vi "Read Forces.vi"(8 "error in":errorcluster, 10 "index":i32, 11 "CIFCorePlugin in":refnum<class "CIFCorePlugin.lvclass">) -> (0 "error out":errorcluster, 2 "Force":T1 {"Force Data" format="%x"}, 3 "CIFCorePlugin out":refnum<class "CIFCorePlugin.lvclass">)   [LabVIEW 2021, in "CIFCorePlugin.lvclass"]
uses:
  CIFCorePlugin.lvclass
  Common/Typedef/Channel Force Data.ctl
  CIFCorePlugin.lvclass/CIFCorePlugin.ctl
  Common/CIFCoreCommon.lvlib
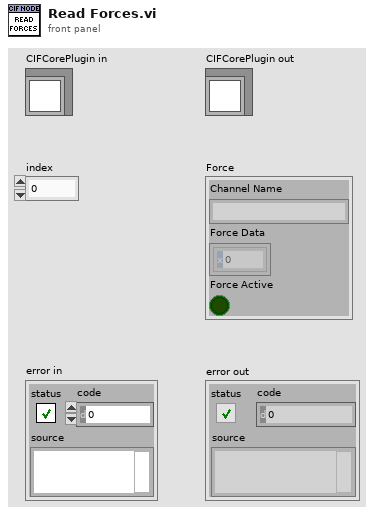
[diagram p1: front panel]
types:
  T1 = typedef "CIFCoreCommon.lvlib/Channel Force Data.ctl" = cluster{"Channel Name":string, "Force Data":u8[], "Force Active":bool}
  T2 = typedef "CIFCorePlugin.lvclass/gRPC to Main DVR.ctl" = refnum<data-value>
  T3 = typedef "CIFCoreCommon.lvlib/gRPC to Main Data.ctl" = cluster{"Config Data":variant, "Connections":T4[], "Forces":T1[], "Clock Conversion":T5, "Publisher Instance":T7}
  T4 = typedef "CIFCoreCommon.lvlib/Channel Connection Data.ctl" = cluster{"Publisher Name":string, "Subscriber Name":string, "Connection Data":u8[]}
  T5 = typedef "Time_CIF_U.lvlib/Clock Conversion Map.ctl" = map{u8, cluster{"Last Reset":i64, "Offset Pair":T6, "Slope":dbl, "1/Slope":dbl}}
  T6 = typedef "Time_CIF_U.lvlib/Timestamp Pair.ctl" = cluster{"System Time":i64, "External Time":i64}
  T7 = typedef "CIFCoreCommon.lvlib/FIFO Publisher.ctl" = cluster{"Publisher Name":string, "New FIFO Instance Config":T8}
  T8 = typedef "ChannelCommon.lvlib/New FIFO Instance Configuration.ctl" = cluster{"Backpressure":bool, "Bytes/Message Override":u32, "Messages/FIFO Override":u32, "Custom Data":u8[]}
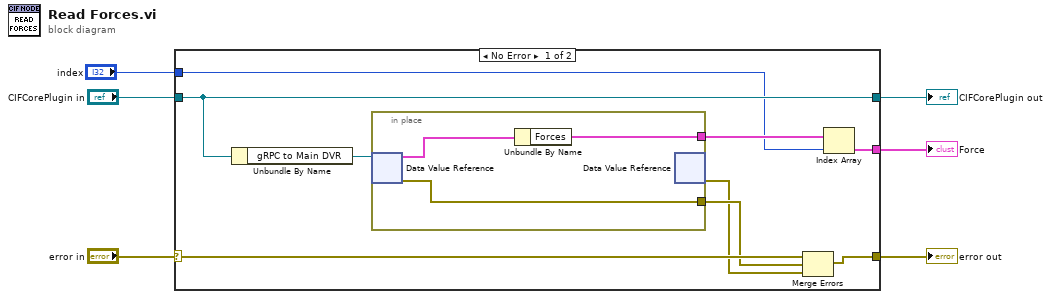
[diagram p0: block diagram]
diagram:
  n1 = case shown="No Error" "error in" {
    selector: "error in" -> [w13 w20]
    tunnel: [w10 w20] -> w5
    tunnel: "CIFCorePlugin in" -> [w15 w19]
    tunnel: [w15 w19] -> w3
    tunnel: [w8 _] -> w2
    tunnel: "index" -> [w7 _]
    frame No Error {
      n2 = Unbundle By Name(w15) -> ("gRPC to Main DVR"=w14:T2)
      n3 = in-place {
        in-place-border: [w17] -> w9
        in-place-border: [w16] -> w12
        n4 = in-place-dvr #1(w14) -> (w18:T3, w16:errorcluster)
        n5 = Unbundle By Name(w18) -> ("Forces"=w17:T1[])
        n6 = in-place-dvr #1() -> (w11:errorcluster)  [unwired: 1 in, 1 out]
      }
      n7 = Merge Errors(w13, w12, w11) -> (w10:errorcluster)
      n8 = Index Array(array=w9, index=w7) -> (element=w8:T1)
    }
    frame Error {
    }
  }
  "error out" <- w5
  "CIFCorePlugin out" <- w3
  "Force" <- w2
